vi "DQMH Tester Prepare hse-appl.vi"(8 "error in":errorcluster, 11 "RT App Name or Path":string) -> (0 "error out":errorcluster, 1 "global shutdown event":refnum<user-event>, 2 "Logging Event":refnum<user-event>, 3 "Started?":bool)   [LabVIEW 2022 SP3, in "hse-dqmh.lvlib"]
doc: "If the hse-application class is not running, queries the user for the path of the containing application and instantiates the hse-appl class. Returns if it did load the class.\n\nHSE projects follow this folder structure:\n /APP-NAME_Config .......... Configuration Files\n /APP-NAME_Data .............. Measured and Other Data\n /APP-NAME_Source .......... LabVIEW Sources\n /APP-NAME ........................ Compiled Application\n\nThe hse-application:ApplicationInit.VI expects the \"APP-NAME_Source\" folder and the \"application name\", and processes these to automatically find the \"_Config\" and \"_Data\" directories.\n\nREAL-TIME: As the configuration directory on real-time systems always needs to reside at \"C:\\<Project Name>_Config\\\", and as it tedious (embedded UI) or impossible (no embedded UI) to enter the path, it can be supplied via the optional Real-Time App Name string input.\n\nIf this VI is used outside of the normal application scope (e.g. in a unit test with a seperate LV project) you can provide the absolute path to the app source folder to \"RT App Name or Path\".\n\n____\nHAMPEL SOFTWARE ENGINEERING v3.8.0 (2023-12-18 14:41)"
uses:
  hse-dqmh.lvlib
  hse-application/hse-application.lvclass
  <vilib>/Hampel Software Engineering/HSE Logger/hse-logger.lvlib
  <vilib>/Hampel Software Engineering/HSE Logger/Handler/UserEventHandler/UserEventHandler.lvclass
  <vilib>/Hampel Software Engineering/HSE Logger/LogLevel.ctl
  C:/Program Files (x86)/National Instruments/LabVIEW 2020/vi.lib/Hampel Software Engineering/HSE Logger/Handler/Handler.lvclass
  <vilib>/Hampel Software Engineering/HSE Logger/LogRecord/LogRecord.lvclass
panel:
  # "If the hse-application class is not running, queries the user for the path of the containing application and instantiates the hse-appl class. Returns if it did load the class.\n\nHSE projects follow this folder structure:\n    /APP-NAME_Config .......... Configuration Files\n    /APP-NAME_Data .............. Measured and Other Data\n    /APP-NAME_Source .......... LabVIEW Sources\n    /APP-NAME ........................ Compiled Application\n\nThe hse-application:ApplicationInit.VI expects the \"APP-NAME_Source\" folder and the \"application name\", and processes these to automatically find the \"_Config\" and \"_Data\" directories.\n\nREAL-TIME: As the configuration directory on real-time systems always needs to reside at \"C:\\<Project Name>_Config\\\", and as it tedious (embedded UI) or impossible (no embedded UI) to enter the path, it can be supplied via the optional Real-Time App Name string input."
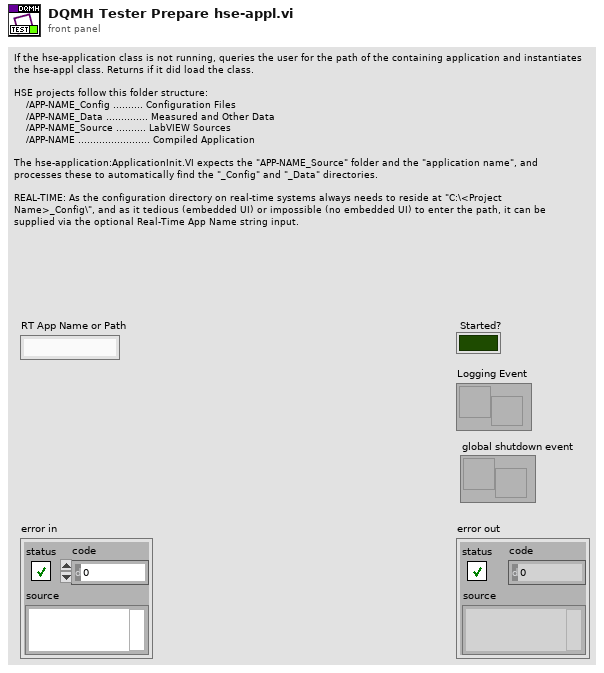
[diagram p1: front panel]
types:
  T1 = typedef "hse-logger.lvlib/LogLevel.ctl" = enum16{"DEBUG", "INFO", "WARNING", "ERROR", "CRITICAL"}
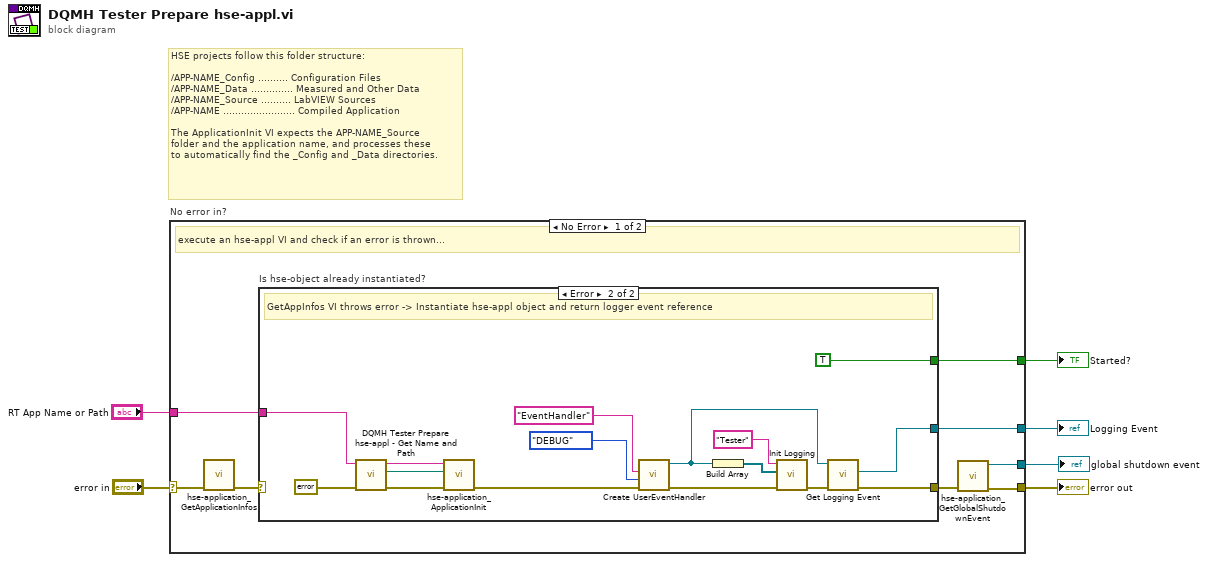
[diagram p0: block diagram]
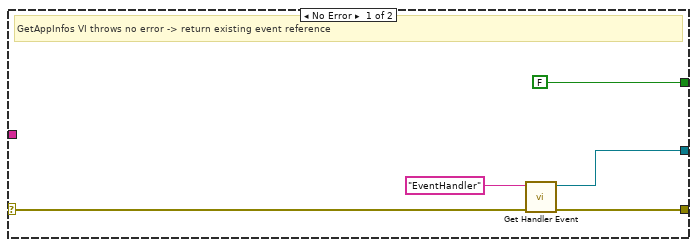
[diagram p2: hidden frame]
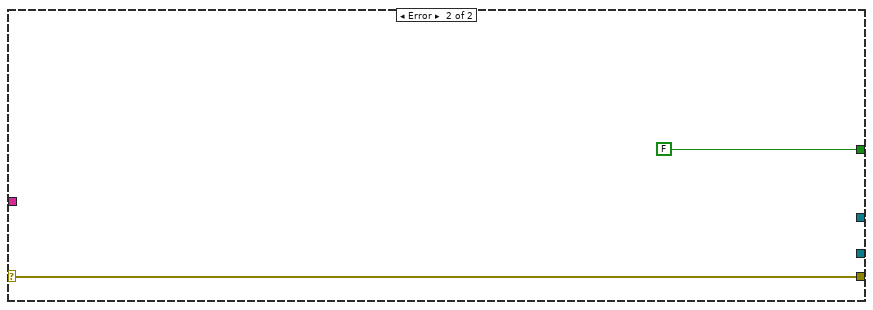
[diagram p3: hidden frame]
diagram:
  # "HSE projects follow this folder structure:\n\n/APP-NAME_Config .......... Configuration Files\n/APP-NAME_Data .............. Measured and Other Data\n/APP-NAME_Source .......... LabVIEW Sources\n/APP-NAME ........................ Compiled Application\n\nThe ApplicationInit VI expects the APP-NAME_Source\nfolder and the application name, and processes these\nto automatically find the _Config and _Data directories."
  n1 = case "No error in?" shown="No Error" "error in" {
    selector: "error in" -> [w14 w37]
    tunnel: [w9 w37] -> w6
    tunnel: [w12 FALSE] -> w4
    tunnel: [w11 _] -> w3
    tunnel: [w8 _] -> w2
    tunnel: "RT App Name or Path" -> [w7 _]
    frame No Error {
      # "execute an hse-appl VI and check if an error is thrown..."
      n2 = call "hse-application_GetApplicationInfos.vi"("error in"=w14) -> ("error out"=w13:errorcluster)  [unwired: 7 in, 3 out]
      n3 = case "Is hse-object already instantiated?" shown="Error" w13 {
        selector: w13 -> [w17 _]
        tunnel: [w16 w28] -> w10
        tunnel: [FALSE TRUE] -> w12
        tunnel: [w15 w26] -> w11
        tunnel: w7 -> [_ w22]
        frame No Error {
          # "GetAppInfos VI throws no error -> return existing event reference"
          n4 = call <vilib>:"Get Handler Event.vi"("error in"=w17, "Name"="EventHandler") -> ("error out"=w16:errorcluster, "Logging Event"=w15:refnum<user-event>)  [unwired: 8 in]
        }
        frame Error {
          # "GetAppInfos VI throws error -> Instantiate hse-appl object and return logger event reference"
          n5 = call "DQMH Tester Prepare hse-appl - Get Name and Path.vi"("error in"=errorcluster {"status"=FALSE, "code"=0, "source"=""} ("error constant"), "RT App Name or Path"=w22) -> ("error out"=w35:errorcluster, "Project Path"=w24:path, "Project Name"=w25:string)  [unwired: 7 in]
          n6 = call "hse-application_ApplicationInit.vi"("error in"=w35, "Project Folder"=w24, "Project Name"=w25) -> ("error out"=w33:errorcluster)  [unwired: 8 in]
          n7 = call <vilib>:"Create UserEventHandler.vi"("error in"=w33, "Level"=LogLevel."DEBUG", "Name"="EventHandler") -> ("error out"=w32:errorcluster, "UserEventHandler out"=w27:refnum<class "UserEventHandler.lvclass">)  [unwired: 7 in]
          n8 = Build Array(w27) -> (w34:refnum<class "UserEventHandler.lvclass">[])
          n9 = call <vilib>:"Init Logging.vi"("error in"=w32, "Handlers"=w34, "Name"="Tester") -> ("error out"=w29:errorcluster)  [unwired: 8 in]
          n10 = call-dynamic "Get Logging Event.vi"("error in"=w29, "UserEventHandler in"=w27) -> ("error out"=w28:errorcluster, "Logging Event"=w26:refnum<user-event>)  [unwired: 7 in, 1 out]
        }
      }
      n11 = call "hse-application_GetGlobalShutdownEvent.vi"("error in"=w10) -> ("error out"=w9:errorcluster, "global shutdown event"=w8:refnum<user-event>)  [unwired: 9 in]
    }
    frame Error {
    }
  }
  "error out" <- w6
  "Started?" <- w4
  "Logging Event" <- w3
  "global shutdown event" <- w2
